vi "VisWindowMinimized.vi"(8 "error in (no error)":errorcluster, 9 "Window Minimized?":bool, 10 "Module Name":string) -> (0 "error out":errorcluster)   [LabVIEW 2018, in "Visualization.lvlib" / "VisualizeBase.lvclass"]
uses:
  VisualizeBase.lvclass
  VisBroadcastData.ctl
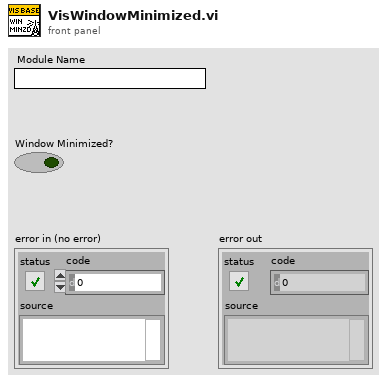
[diagram p1: front panel]
types:
  T1 = typedef "Visualization.lvlib/VisualizeBase.lvclass/VisBroadcastData.ctl" = cluster{"Module Name":string, "Data":variant}
  T2 = typedef "Visualization.lvlib/VisualizeBase.lvclass/VisBroadcastEvents.ctl" = cluster{"WindowMinimized":refnum<user-event>, "WindowClosed":refnum<user-event>, "DidStop":refnum<user-event>}
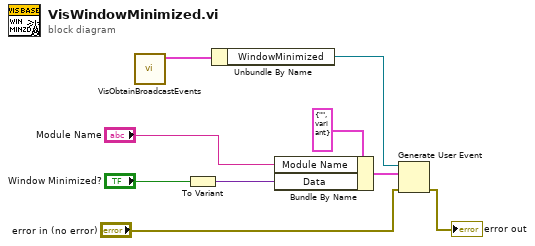
[diagram p0: block diagram]
diagram:
  n1 = call "VisObtainBroadcastEvents.vi"() -> ("VisBroadcastEvents"=w2:T2)  [unwired: 10 in, 1 out]
  n2 = To Variant(anything="Window Minimized?") -> (Variant=w7:variant)
  n3 = Unbundle By Name(w2) -> ("WindowMinimized"=w9:refnum<user-event>)
  n4 = Bundle By Name(cluster=T1 {"Module Name"="", "Data"=variant} ("clBroadcast"), "Module Name"="Module Name", "Data"=w7) -> (w6:T1)
  n5 = Generate User Event(user event=w9, event data cluster=w6, error in="error in (no error)") -> (error out=→"error out":errorcluster)  [unwired: 1 in, 1 out]
